vi "Actor Core.vi"(8 "error in":errorcluster, 11 "Nested in":refnum<class "DataLoggerUI.lvclass">) -> (0 "error out":errorcluster, 3 "Actor out":refnum<class "Actor.lvclass">)   [LabVIEW 2020, in "DataLoggerUI.lvlib" / "DataLoggerUI.lvclass"]
doc: "(<B>Filename</B>: Actor Framework.lvlib:Actor.lvclass:Actor Core.vi)\n\nReceives messages to the actor, reacts to them, and initiates any error handling that may shut the actor down.\n\nDescendant classes may override this VI to append parallel tasks for the actor to complete while it handles messages. Overrides use the Call Parent Method node."
uses:
  DataLoggerUI.lvclass
  C:/Program Files/National Instruments/LabVIEW 2020/vi.lib/ActorFramework/Actor/Actor.lvclass
  <vilib>/ActorFramework/Actor/Actor.lvclass
  DataLoggerUI.lvclass/DataLoggerUI.ctl
  <vilib>/ActorFramework/Actor/Actor.lvclass/Actor.ctl
  <vilib>/ActorFramework/Message Enqueuer/Message Enqueuer.lvclass/Message Enqueuer.ctl
  Hardware Abstraction Layer/Component/Device/Device/DataExchange.ctl
  Interface/DataListener Messages/OnDataChange Msg/OnDataChange Msg.lvclass/OnDataChange Msg.ctl
  <vilib>/ActorFramework/Message Enqueuer/Init from Existing Queue.vi
  <vilib>/ActorFramework/Message Enqueuer/Enqueue.vi
  Interface/DataListener Messages/OnDataChange Msg/OnDataChange Msg.lvclass
  C:/Program Files/National Instruments/LabVIEW 2020/vi.lib/ActorFramework/Message/Message.lvclass
  <vilib>/ActorFramework/Stop Msg/Stop Msg.lvclass
  <vilib>/ActorFramework/Message Priority Queue/Priority Enqueue.vi
  <vilib>/ActorFramework/Message Enqueuer/Message Enqueuer.lvclass
  Hardware Abstraction Layer/Component/GenericActor/GenericActor/GenericController.lvclass
  Interface/DataListener/DataListener.lvclass
panel:
  in  "Open Button":bool
  in  "File Suffix":string
  in  "Save Path":path
  in  "Alert when finish?":bool
  in  "SingleStack?":bool
  in  "StreamToDisk?":bool
  # "Save Image Mode"
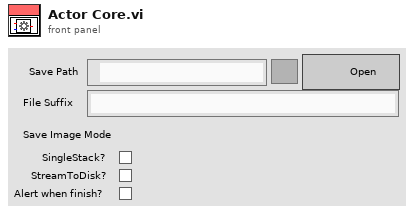
[diagram p1: front panel]
types:
  T1 = cluster{"Stop":refnum<user-event>, "ImagePreview":refnum<user-event>}
  T2 = cluster{"StreamToDisk?":bool, "SingleStack?":bool, "Alert when finish?":bool, "TiffFileFullPath":path, "StreamFileFullPath":path}
  T3 = typedef "DataListener.lvclass/DataExchange.ctl" = cluster{"Source":string, "Destination":string, "Description":string, "value":variant}
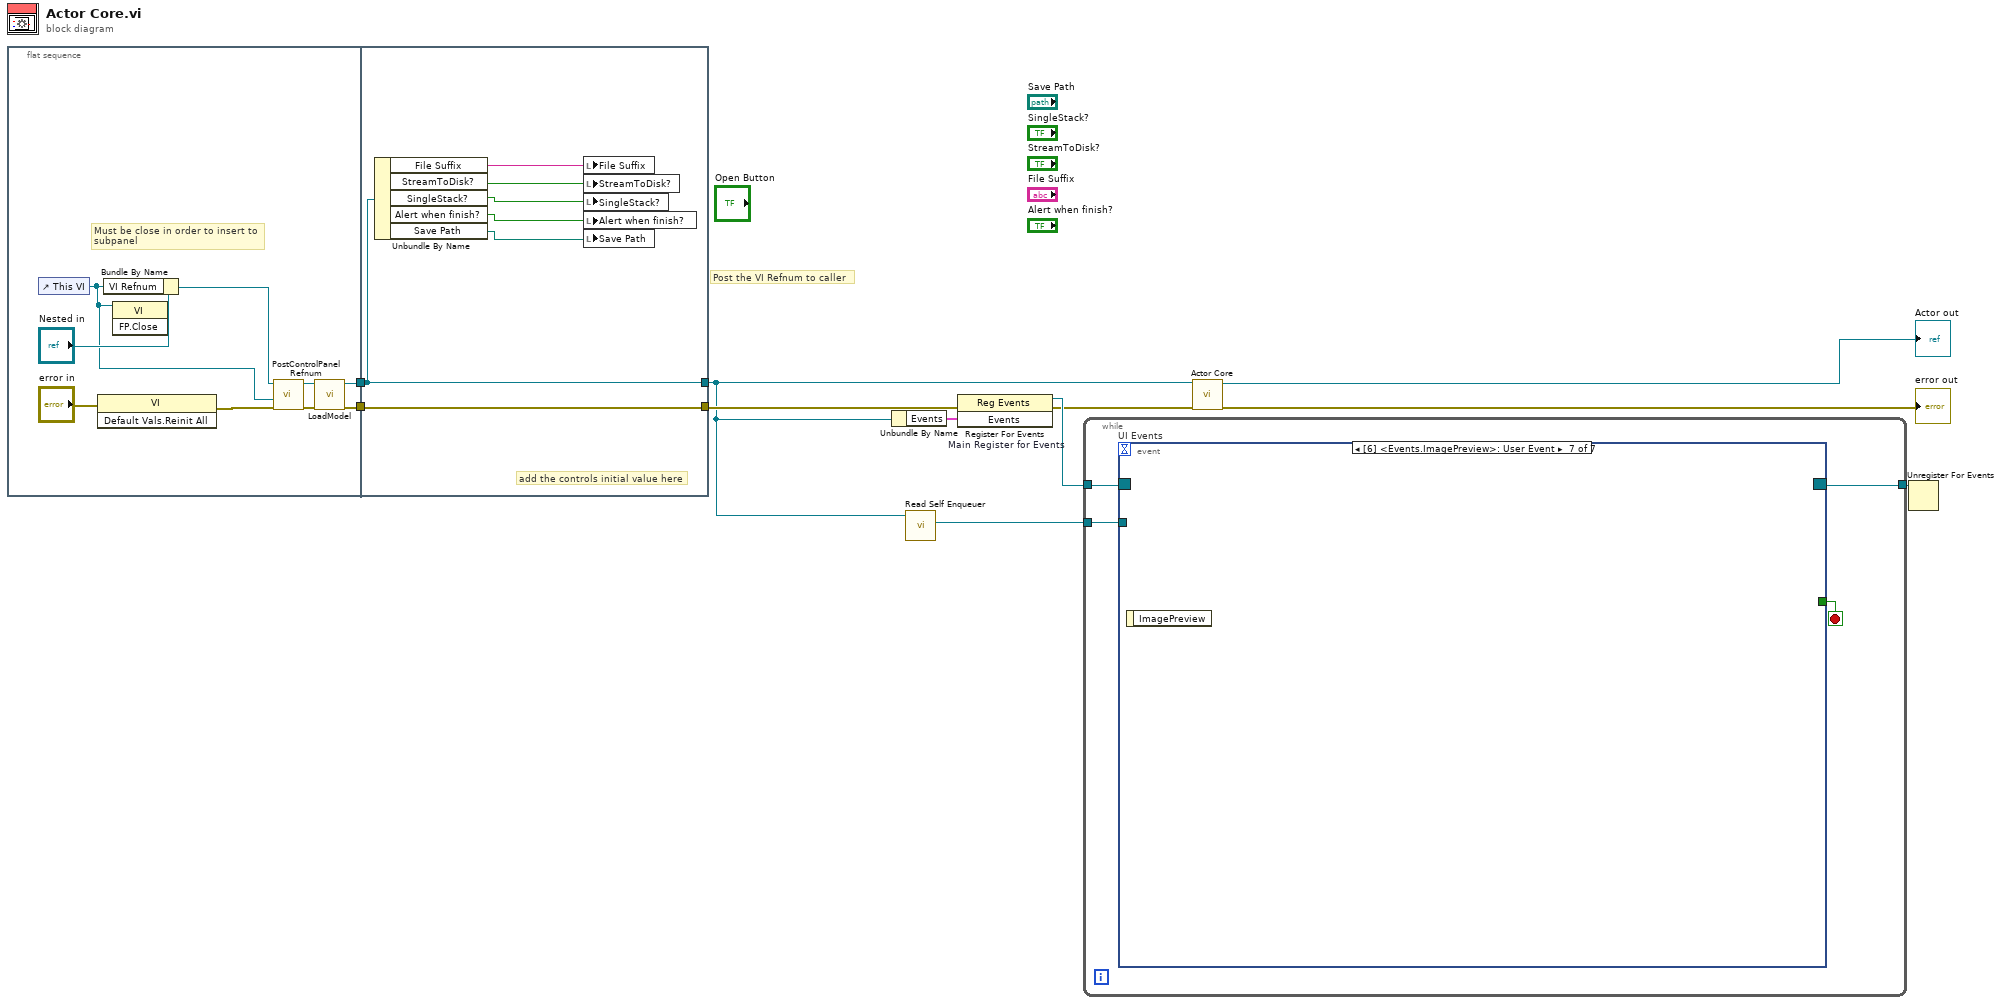
[diagram p0: block diagram]
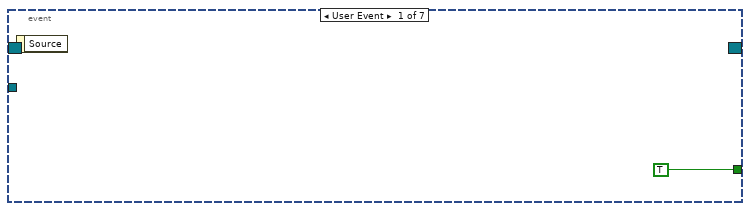
[diagram p2: hidden frame]
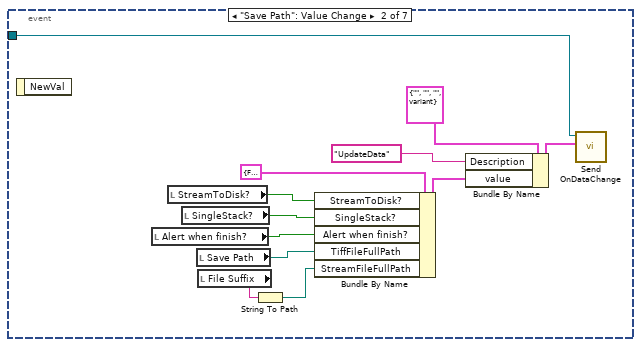
[diagram p3: hidden frame]
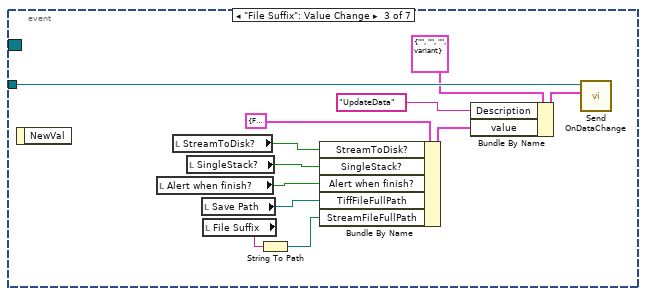
[diagram p4: hidden frame]
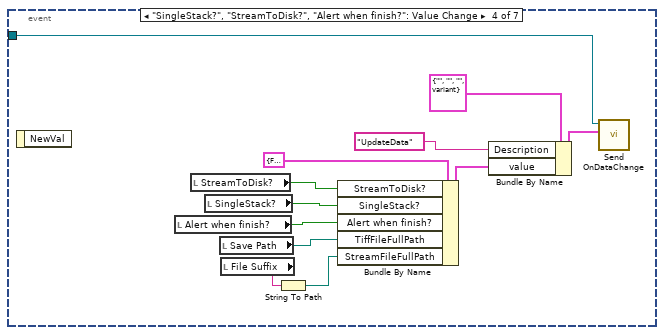
[diagram p5: hidden frame]
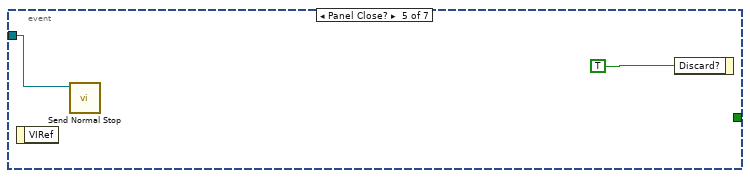
[diagram p6: hidden frame]
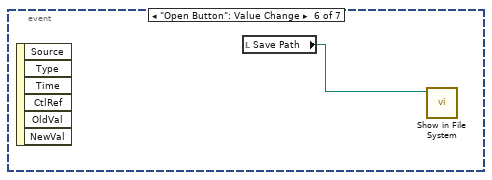
[diagram p7: hidden frame]
diagram:
  # "Post the VI Refnum to caller"
  n1 = flat-sequence {
    tunnel: [w14] -> w5
    tunnel: [w12] -> w4
    tunnel: [w26] -> w2
    tunnel: [w27] -> w3
    tunnel: w5 -> [w27]
    tunnel: w4 -> [w26]
    frame #0 {
      # "Must be close in order to insert to\nsubpanel"
      n2 = control-ref of="This VI"() -> (w15:refnum<vi>)
      n3 = invoke class="VI" method="Default Vals.Reinit All"(error in="error in") -> (error out=w18:errorcluster)  [unwired: 2 in, 2 out]
      n4 = Bundle By Name(cluster="Nested in", "VI Refnum"=w15) -> (w16:refnum<class "DataLoggerUI.lvclass">)
      n5 = invoke class="VI" method="FP.Close"(reference=w15) -> ()  [unwired: 2 in, 3 out]
      n6 = call-dynamic "PostControlPanelRefnum.vi"("error in (no error)"=w18, "VI Refnum"=w15, "GRMActor in"=w16) -> ("error out"=w17:errorcluster, "GRMActor out"=w13:refnum<class "DataLoggerUI.lvclass">)  [unwired: 7 in]
      n7 = call-dynamic "LoadModel.vi"("error in (no error)"=w17, "GRMActor in"=w13) -> ("error out"=w14:errorcluster, "GRMActor out"=w12:refnum<class "DataLoggerUI.lvclass">)  [unwired: 8 in]
    }
    frame #1 {
      # "add the controls initial value here"
      n8 = Unbundle By Name(w26) -> ("File Suffix"=w25:string, "StreamToDisk?"=w24:bool, "SingleStack?"=w23:bool, "Alert when finish?"=w22:bool, "Save Path"=w21:path)
      n9 = local write "File Suffix"(w25) -> ()
      n10 = local write "StreamToDisk?"(w24) -> ()
      n11 = local write "SingleStack?"(w23) -> ()
      n12 = local write "Alert when finish?"(w22) -> ()
      n13 = local write "Save Path"(w21) -> ()
    }
  }
  n14 = Unbundle By Name(w2) -> ("Events"=w8:T1)
  n15 = call <vilib>:"Read Self Enqueuer.vi"("Actor"=w2) -> ("Self Enqueuer"=w1:refnum<class "Message Enqueuer.lvclass">)  [unwired: 10 in]
  n16 = register-events "Main Register for Events"(error in=w3, w8) -> (reference out=w9:refnum<event-registration>, error out=w6:errorcluster)  [unwired: 1 in]
  n17 = while {
    tunnel: w9 -> [w31]
    tunnel: [w29] -> w7
    tunnel: w1 -> [w28]
    stop <- w30 stop-if-true
    n18 = event "UI Events" shown="[6] <Events.ImagePreview>: User Event" {
      selector: w31 -> [_ _ _ _ _ _ _]
      dyn-events: [_ _ _ _ _ _ _] -> w29
      timeout: _ -> [_ _ _ _ _ _ _]
      tunnel: [TRUE _ _ _ _ _ _] -> w30
      tunnel: w28 -> [_ w33 w56 w57 w69 _ _]
      event User Event {
        n19 = event-data() -> ()  [unwired: 1 in, 1 out]
      }
      event "Save Path": Value Change {
        n20 = event-data() -> ()  [unwired: 1 in, 1 out]
        n21 = local read "Alert when finish?"() -> (w37:bool)
        n22 = local read "StreamToDisk?"() -> (w39:bool)
        n23 = local read "SingleStack?"() -> (w38:bool)
        n24 = local read "Save Path"() -> (w36:path)
        n25 = local read "File Suffix"() -> (w35:string)
        n26 = String To Path(string=w35) -> (path=w34:path)
        n27 = Bundle By Name(cluster=T2 {"StreamToDisk?"=FALSE, "SingleStack?"=FALSE, "Alert when finish?"=FALSE, "TiffFileFullPath"=path "", "StreamFileFullPath"=path ""} ("Images Saving"), "StreamToDisk?"=w39, "SingleStack?"=w38, "Alert when finish?"=w37, "TiffFileFullPath"=w36, "StreamFileFullPath"=w34) -> (w40:T2)
        n28 = Bundle By Name(cluster=T3 {"Source"="", "Destination"="", "Description"="", "value"=variant} ("DataExchange"), "Description"="UpdateData", "value"=w40) -> (w43:T3)
        n29 = call "Send OnDataChange.vi"("DataExchange"=w43, "Message Enqueuer"=w33) -> ()  [unwired: 8 in, 2 out]
      }
      event "File Suffix": Value Change {
        n30 = event-data() -> ()  [unwired: 1 in, 1 out]
        n31 = local read "Alert when finish?"() -> (w48:bool)
        n32 = local read "StreamToDisk?"() -> (w50:bool)
        n33 = local read "SingleStack?"() -> (w49:bool)
        n34 = local read "Save Path"() -> (w47:path)
        n35 = local read "File Suffix"() -> (w46:string)
        n36 = String To Path(string=w46) -> (path=w45:path)
        n37 = Bundle By Name(cluster=T2 {"StreamToDisk?"=FALSE, "SingleStack?"=FALSE, "Alert when finish?"=FALSE, "TiffFileFullPath"=path "", "StreamFileFullPath"=path ""} ("Images Saving"), "StreamToDisk?"=w50, "SingleStack?"=w49, "Alert when finish?"=w48, "TiffFileFullPath"=w47, "StreamFileFullPath"=w45) -> (w51:T2)
        n38 = Bundle By Name(cluster=T3 {"Source"="", "Destination"="", "Description"="", "value"=variant} ("DataExchange"), "Description"="UpdateData", "value"=w51) -> (w54:T3)
        n39 = call "Send OnDataChange.vi"("DataExchange"=w54, "Message Enqueuer"=w56) -> ()  [unwired: 8 in, 2 out]
      }
      event "SingleStack?", "StreamToDisk?", "Alert when finish?": Value Change {
        n40 = event-data() -> ()  [unwired: 1 in, 1 out]
        n41 = local read "Alert when finish?"() -> (w64:bool)
        n42 = local read "StreamToDisk?"() -> (w66:bool)
        n43 = local read "SingleStack?"() -> (w65:bool)
        n44 = local read "Save Path"() -> (w63:path)
        n45 = local read "File Suffix"() -> (w62:string)
        n46 = String To Path(string=w62) -> (path=w61:path)
        n47 = Bundle By Name(cluster=T2 {"StreamToDisk?"=FALSE, "SingleStack?"=FALSE, "Alert when finish?"=FALSE, "TiffFileFullPath"=path "", "StreamFileFullPath"=path ""} ("Images Saving"), "StreamToDisk?"=w66, "SingleStack?"=w65, "Alert when finish?"=w64, "TiffFileFullPath"=w63, "StreamFileFullPath"=w61) -> (w67:T2)
        n48 = Bundle By Name(cluster=T3 {"Source"="", "Destination"="", "Description"="", "value"=variant} ("DataExchange"), "Description"="UpdateData", "value"=w67) -> (w68:T3)
        n49 = call "Send OnDataChange.vi"("DataExchange"=w68, "Message Enqueuer"=w57) -> ()  [unwired: 8 in, 2 out]
      }
      event Panel Close? {
        n50 = event-data() -> ()  [unwired: 1 in, 1 out]
        n51 = call <vilib>:"Send Normal Stop.vi"("Message Enqueuer"=w69) -> ()  [unwired: 10 in, 1 out]
        n52 = event-data("Discard?"=TRUE) -> ()  [unwired: 1 in, 1 out]
      }
      event "Open Button": Value Change {
        n53 = event-data() -> ()  [unwired: 1 in, 6 out]
        n54 = local read "Save Path"() -> (w71:path)
        n55 = call <vilib>:"Show in File System.vi"("file or directory path"=w71) -> ()  [unwired: 10 in, 1 out]
      }
      event User Event {
        n56 = event-data() -> ()  [unwired: 1 in, 1 out]
      }
    }
  }
  n57 = call-parent "Actor Core.vi"("error in"=w6, "GenericController in"=w2) -> ("error out"=→"error out":errorcluster, "Actor out"=→"Actor out":refnum<class "Actor.lvclass">)  [unwired: 8 in]
  n58 = Unregister For Events(event registration refnum=w7) -> ()  [unwired: 1 in, 1 out]
